vi "Queue Driver.vi"(0 "States and data":cluster{"State":string, "Data":variant}[](array[cluster]), 2 "Name":string, 11 "Error in":errorcluster, 13 "Queue operations":T1) -> (4 "Dequeue data":cluster{"State":string, "Data":variant}, 15 "Error out":errorcluster)   [LabVIEW 2020, in "Automated teller machine.lvlib"]
uses:
  Automated teller machine.lvlib
  Typedefs/Queue driver operations.ctl
  Typedefs/Queue data.ctl
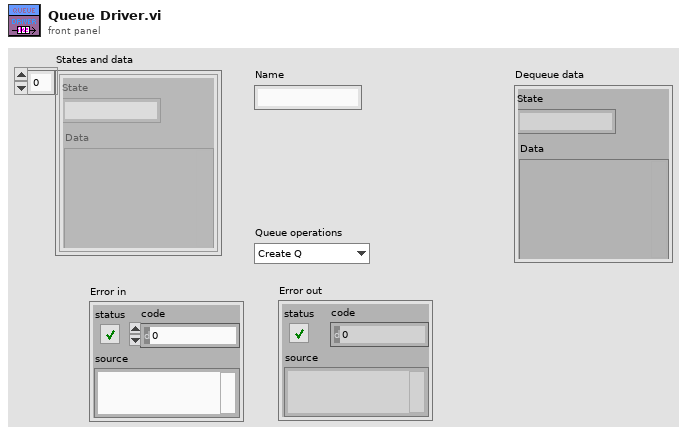
[diagram p1: front panel]
types:
  T1 = typedef "Automated teller machine.lvlib/Queue driver operations.ctl" = enum16{"Create Q", "Enqueue", "Enstack", "Dequeue", "Flush", "Release"}
  T2 = typedef "Automated teller machine.lvlib/Queue data.ctl" = cluster{string, variant}
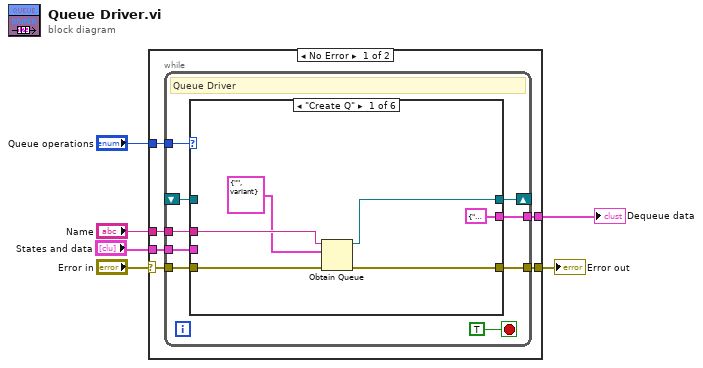
[diagram p0: block diagram]
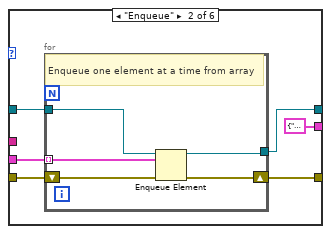
[diagram p2: hidden frame]
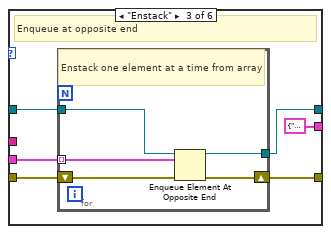
[diagram p3: hidden frame]
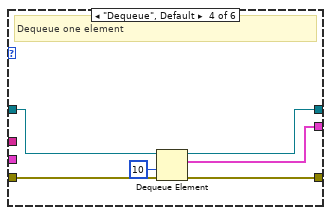
[diagram p4: hidden frame]
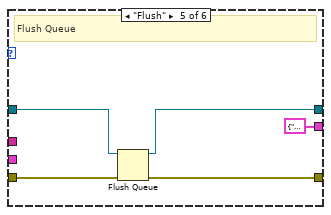
[diagram p5: hidden frame]
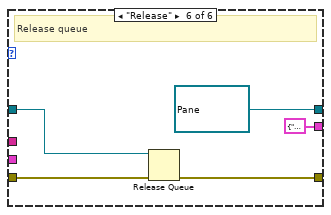
[diagram p6: hidden frame]
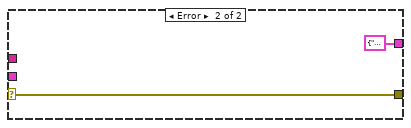
[diagram p7: hidden frame]
diagram:
  n1 = case shown="No Error" "Error in" {
    selector: "Error in" -> [w11 w67]
    tunnel: [w12 w67] -> w5
    tunnel: "Queue operations" -> [w10 _]
    tunnel: "Name" -> [w9 _]
    tunnel: "States and data" -> [w8 _]
    tunnel: [w7 cluster{string, variant} {"", variant}] -> w1
    frame No Error {
      n2 = while {
        tunnel: [w20] -> w12
        tunnel: w11 -> [w19]
        tunnel: w10 -> [w18]
        tunnel: w9 -> [w17]
        tunnel: w8 -> [w16]
        shift-right: [w15] -> _
        shift-left: _ -> [w14]
        tunnel: [w13] -> w7
        stop <- TRUE stop-if-true
        # "Queue Driver"
        n3 = case shown="\"Create Q\"" w18 {
          tunnel: [w26 w32 w43 w54 w59 w64] -> w20
          tunnel: w19 -> [w27 w33 w44 w55 w60 w65]
          tunnel: w17 -> [w25 _ _ _ _ _]
          tunnel: w16 -> [_ w29 w40 _ _ _]
          tunnel: [w23 w31 w41 w53 w57 refnum<queue> refnum ("queue out")] -> w15
          tunnel: w14 -> [_ w30 w42 w52 w58 w63]
          tunnel: [cluster{string, variant} {"", variant} cluster{string, variant} {"", variant} cluster{string, variant} {"", variant} w50 cluster{string, variant} {"", variant} cluster{string, variant} {"", variant}] -> w13
          frame "Create Q" {
            n4 = Obtain Queue(name (unnamed)=w25, element data type=T2 {"", variant}, error in (no error)=w27) -> (queue out=w23:refnum<queue>, error out=w26:errorcluster)  [unwired: 2 in, 1 out]
          }
          frame "Enqueue" {
            n5 = for {
              tunnel: [w36] -> w31
              tunnel: w30 -> [w35]
              shift-right: [w37] -> w32
              shift-left: w33 -> [w38]
              tunnel: w29 -> [w34] mode=indexing
              # "Enqueue one element at a time from array"
              n6 = Enqueue Element(queue=w35, element=w34, error in (no error)=w38) -> (queue out=w36:refnum<queue>, error out=w37:errorcluster)  [unwired: 1 in, 1 out]
            }
          }
          frame "Enstack" {
            # "Enqueue at opposite end"
            n7 = for {
              tunnel: w42 -> [w47]
              tunnel: [w46] -> w41
              shift-right: [w48] -> w43
              shift-left: w44 -> [w49]
              tunnel: w40 -> [w45] mode=indexing
              # "Enstack one element at a time from array"
              n8 = Enqueue Element At Opposite End(queue=w47, element=w45, error in (no error)=w49) -> (queue out=w46:refnum<queue>, error out=w48:errorcluster)  [unwired: 1 in, 1 out]
            }
          }
          frame "Dequeue", Default {
            # "Dequeue one element"
            n9 = Dequeue Element(queue=w52, timeout in ms (-1)=10, error in (no error)=w55) -> (queue out=w53:refnum<queue>, element=w50:cluster{string, variant}, error out=w54:errorcluster)  [unwired: 1 out]
          }
          frame "Flush" {
            # "Flush Queue"
            n10 = Flush Queue(queue=w58, error in (no error)=w60) -> (queue out=w57:refnum<queue>, error out=w59:errorcluster)  [unwired: 1 out]
          }
          frame "Release" {
            # "Release queue"
            n11 = Release Queue(queue=w63, error in (no error)=w65) -> (error out=w64:errorcluster)  [unwired: 1 in, 2 out]
          }
        }
      }
    }
    frame Error {
    }
  }
  "Error out" <- w5
  "Dequeue data" <- w1
